vi "HistogramMeasurement.vi"(6 "Histogram minimum / ns (0)":dbl, 7 "Histogram maximum / ns (100)":dbl=100.0, 8 "error in (no error)":errorcluster, 9 "Number of bins (50)":i32=50, 10 "Time to measure (1000)":i32=1000, 11 "VISA resource name":refnum<visa-resource-name>) -> (0 "error out":errorcluster, 1 "Counts":dbl[](array[numeric]), 2 "Times / ns":dbl[](array[numeric]), 3 "VISA resource name out":refnum<visa-resource-name>)   [LabVIEW 2017, in "GP22_TDC_Arduinoed.lvlib"]
doc: "Configure the GP22 for a series of measurments. The microprocessor will bin these into a histogram using the passed parameters. This method is quicker than returning all data and letting labview do the binning."
uses:
  GP22_TDC_Arduinoed.lvlib
panel:
  out "XY Graph":cluster{"Array":dbl[], dbl[]}(graph)
  out "read buffer":string
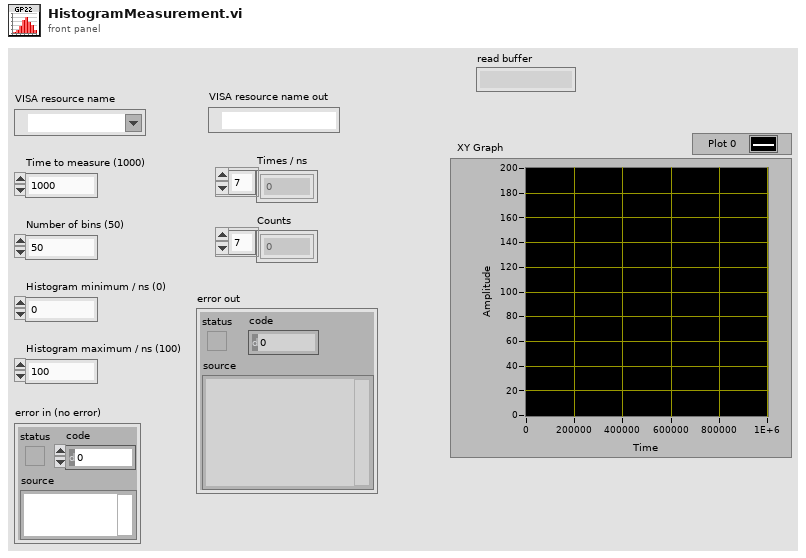
[diagram p1: front panel]
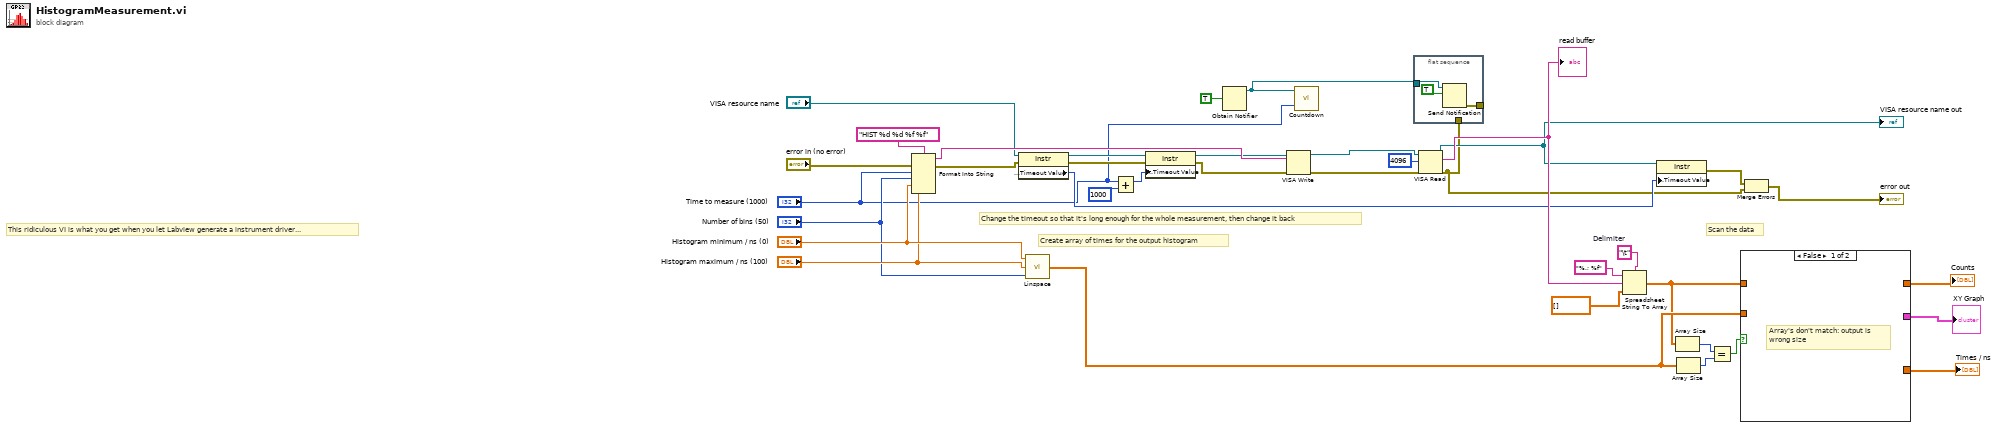
[diagram p0: block diagram]
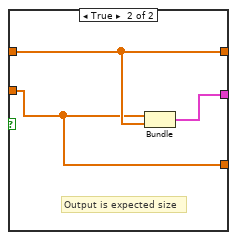
[diagram p2: hidden frame]
diagram:
  w33 = "\t"  # Delimiter
  # "Scan the data"
  # "Change the timeout so that it's long enough for the whole measurement, then change it back"
  # "Create array of times for the output histogram"
  # "This ridiculous VI is what you get when you let Labview generate a instrument driver..."
  n1 = Format Into String(format string="HIST %d %d %f %f", error in="error in (no error)", "Time to measure (1000)", "Number of bins (50)", "Histogram minimum / ns (0)", "Histogram maximum / ns (100)") -> (resulting string=w36:string, error out=w16:errorcluster)  [unwired: 1 in]
  n2 = property class="Instr"(reference="VISA resource name", error in=w16) -> (reference out=w18:refnum<visa-resource-name>, error out=w19:errorcluster, "General Settings:Timeout Value"=w15:u32)
  n3 = call "Linspace.vi"("NumElements"="Number of bins (50)", "End"="Histogram maximum / ns (100)", "Start"="Histogram minimum / ns (0)") -> ("Array"=w25:dbl[])
  n4 = Add(x="Time to measure (1000)", y=1000) -> (x+y=w21:i32)
  n5 = property class="Instr"(reference=w18, error in=w19, "General Settings:Timeout Value"=w21) -> (reference out=w22:refnum<visa-resource-name>, error out=w4:errorcluster)
  n6 = Obtain Notifier(notification data type=TRUE) -> (notifier out=w3:refnum<notifier>)  [unwired: 3 in, 2 out]
  n7 = VISA Write(VISA resource name=w22, write buffer=w36, error in (no error)=w4) -> (VISA resource name out=w29:refnum<visa-resource-name>, error out=w35:errorcluster)  [unwired: 1 out]
  n8 = call "Countdown.vi"("Time / ms"="Time to measure (1000)", "notifier in"=w3) -> ()  [unwired: 2 in]
  n9 = flat-sequence {
    tunnel: w3 -> [w40]
    tunnel: w1 -> [_]
    tunnel: [w38] -> _
    frame #0 {
      n10 = Send Notification(notification=TRUE, notifier=w40) -> (error out=w38:errorcluster)  [unwired: 1 in, 1 out]
    }
  }
  n11 = VISA Read(VISA resource name=w29, byte count=u32 4096, error in (no error)=w35) -> (VISA resource name out=w23:refnum<visa-resource-name>, read buffer=w30:string, error out=w1:errorcluster)  [unwired: 1 out]
  "VISA resource name out" <- w23
  "read buffer" <- w30
  n12 = Spreadsheet String To Array(delimiter (Tab)=w33, format string="%.; %f", spreadsheet string=w30, array type (2D Dbl)=dbl[] []) -> (array=w24:dbl[])
  n13 = property class="Instr"(reference=w23, "General Settings:Timeout Value"=w15) -> (error out=w14:errorcluster)  [unwired: 1 in, 1 out]
  n14 = Array Size(array=w24) -> (size(s)=w27:i32)
  n15 = Array Size(array=w25) -> (size(s)=w28:i32)
  n16 = Equal?(x=w27, y=w28) -> (x = y?=w12:bool)
  n17 = case shown="False" w12 {
    tunnel: [_ w43] -> w26
    tunnel: w25 -> [_ w41]
    tunnel: w24 -> [_ w42]
    tunnel: [_ w42] -> w11
    tunnel: [_ w41] -> w10
    frame False {
      # "Array's don't match: output is\nwrong size"
    }
    frame True {
      # "Output is expected size"
      n18 = Bundle("Array"=w41, w42) -> (w43:cluster{"Array":dbl[], dbl[]})  [unwired: 1 in]
    }
  }
  "Counts" <- w11
  "XY Graph" <- w26
  "Times / ns" <- w10
  n19 = Merge Errors(w14, w1) -> (→"error out":errorcluster)
